vi "Ejerciciodepractica1.vi"() -> ()   [LabVIEW 2020]
panel:
  in  "Time":i32
  in  "Vi":dbl(knob) scale=0.0..10.0
  in  "C":dbl
  in  "R":dbl
  out "Waveform Chart":dbl(graph)
  out "tiempo":dbl
  out "Vid":dbl
  out "Vic":dbl
  out "Vc":dbl
  in  "stop":bool
  in  "Carga/Descarga":bool
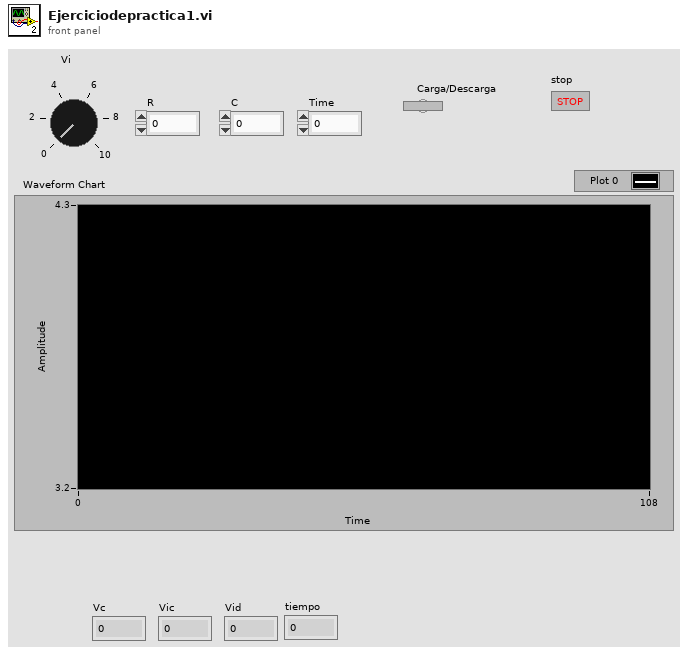
[diagram p1: front panel]
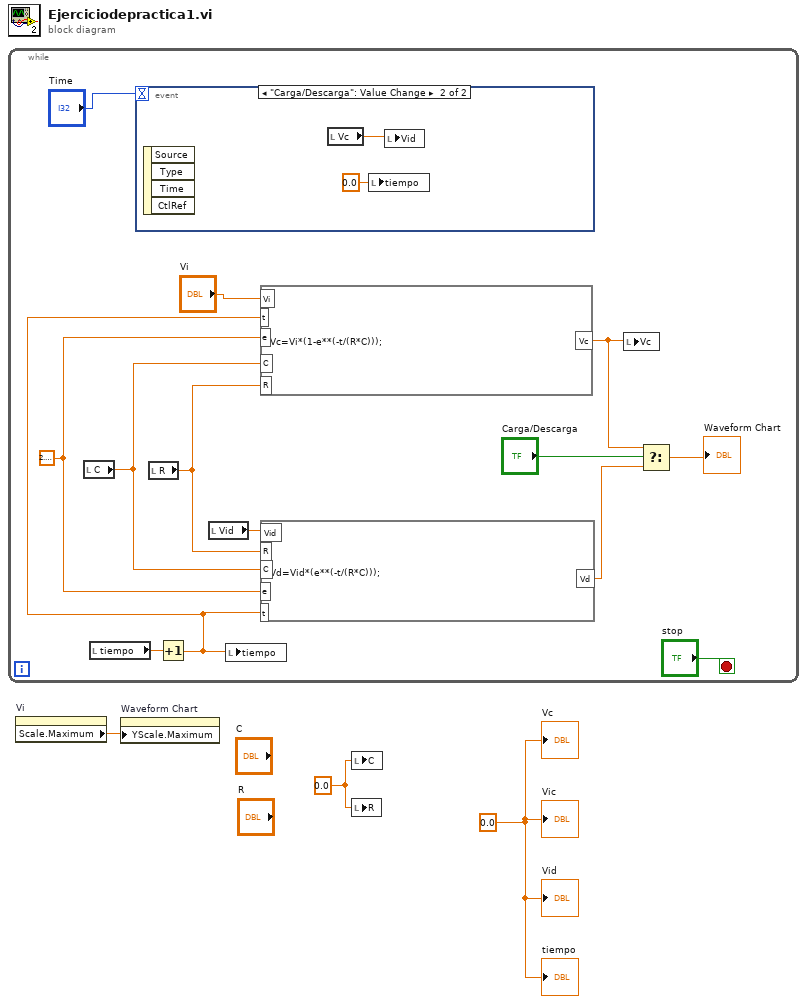
[diagram p0: block diagram]
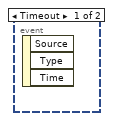
[diagram p2: hidden frame]
diagram:
  w2 = 0.0 ("R")
  w3 = 0.0 ("Vc")
  n1 = while {
    stop <- "stop" stop-if-true
    w15 = 2.718281828459045
    # "Descarga del condensador"
    # "Carga del condensador"
    n2 = local read "C"() -> (w7:dbl)
    n3 = local read "tiempo"() -> (w9:dbl)
    n4 = event shown="[1] \"Carga/Descarga\": Value Change" {
      selector: _ -> [_ _]
      dyn-events: _ -> [_ _]
      timeout: "Time" -> [_ _]
      event Timeout {
        n5 = event-data() -> ()  [unwired: 1 in, 3 out]
      }
      event "Carga/Descarga": Value Change {
        n6 = event-data() -> ()  [unwired: 1 in, 4 out]
        n7 = local read "Vc"() -> (w18:dbl)
        n8 = local write "tiempo"(0.0 ("tiempo")) -> ()
        n9 = local write "Vid"(w18) -> ()
      }
    }
    n10 = local read "R"() -> (w6:dbl)
    n11 = Increment(x=w9) -> (x+1=w8:dbl)
    n12 = local read "Vid"() -> (w14:dbl)
    n13 = local write "tiempo"(w8) -> ()
    n14 = formula code="Vc=Vi*(1-e**(-t/(R*C)));"("Vi"="Vi", "e"=w15, "C"=w7, "t"=w8, "R"=w6) -> ("Vc"=w12:dbl)
    n15 = formula code="Vd=Vid*(e**(-t/(R*C)));"("Vid"=w14, "e"=w15, "R"=w6, "C"=w7, "t"=w8) -> ("Vd"=w13:dbl)
    n16 = local write "Vc"(w12) -> ()
    n17 = Select(t=w12, s="Carga/Descarga", f=w13) -> (s? t:f=→"Waveform Chart":dbl)
  }
  n18 = property on="Vi" class="Knob (strict)"() -> ("Scale.Maximum"=w1:dbl)  [unwired: 2 in, 2 out]
  n19 = property on="Waveform Chart" class="WFChart (strict)"("YScale.Maximum"=w1) -> ()  [unwired: 2 in, 2 out]
  n20 = local write "C"(w2) -> ()
  n21 = local write "R"(w2) -> ()
  "Vc" <- w3
  "Vic" <- w3
  "Vid" <- w3
  "tiempo" <- w3
